vi "Predet_Inject.vi"(11 "Predet Freq (Hz)":dbl=20.0 format="%#_13g") -> ()   [LabVIEW 2017]
uses:
  <vilib>/DAQmx/write.llb/DAQmx Write (Digital 1D Wfm NChan NSamp).vi
  <vilib>/DAQmx/create/channels.llb/DAQmx Create Channel (DO-Digital Output).vi
  <vilib>/DAQmx/configure/timing.llb/DAQmx Timing (Sample Clock).vi
  <vilib>/Waveform/DWDTOps.llb/DWDT Uncompress Digital.vi
  <vilib>/DAQmx/miscellaneous.llb/DAQmx Fill In Error Info.vi
  <resource>/objmgr/daqmx.rc
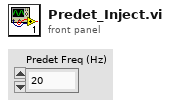
[diagram p1: front panel]
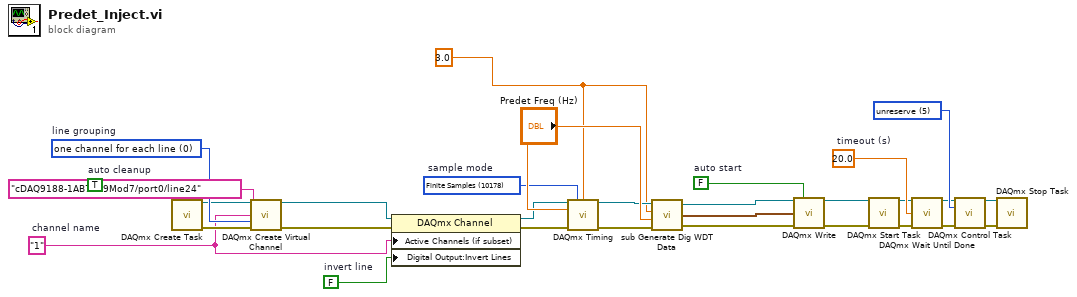
[diagram p0: block diagram]
diagram:
  w1 = 3.0 ("number of samples")
  w29 = 5 items=["verify"=2, "reserve"=4, "commit"=3, "unreserve"=5, "abort"=6] ("action")
  w20 = 10178 items=["Finite Samples"=10178, "Continuous Samples"=10123, "Hardware Timed Single Point"=12522]  # sample mode
  w18 = FALSE  # invert line
  w14 = 0 items=["one channel for each line", "one channel for all lines"]  # line grouping
  w3 = "1"  # channel name
  w12 = TRUE  # auto cleanup
  w10 = 20.0  # timeout (s)
  w4 = FALSE  # auto start
  n1 = call <vilib>:"DAQmx Create Task.vi"("auto cleanup"=w12) -> ("task out"=w13:refnum<k21>, "error out"=w11:errorcluster)  [unwired: 4 in, 9 out]
  n2 = call-poly <vilib>:"DAQmx Create Virtual Channel.vi"("task in"=w13, "lines"=tag "cDAQ9188-1AB7749Mod7/port0/line24", "name to assign"=w3, "line grouping"=w14, "error in"=w11) -> ("task out"=w15:refnum<k21>, "error out"=w16:errorcluster)  [unwired: 9 out]
  n3 = property class="DAQmx Channel"(reference=w15, error in=w16, "Active Channels (if subset)"=w3, "Digital Output:Invert Lines"=w18) -> (reference out=w19:refnum<k21>, error out=w17:errorcluster)
  n4 = call-poly <vilib>:"DAQmx Timing.vi"("task/channels in"=w19, "sample mode"=w20, "samples per channel"=w1, "rate"="Predet Freq (Hz)", "error in"=w17) -> ("task out"=w21:refnum<k21>, "error out"=w22:errorcluster)  [unwired: 2 in, 7 out]
  n5 = call <vilib>:"sub Generate Dig WDT Data.vi"("task in"=w21, "number of samples"=w1, "update rate"="Predet Freq (Hz)", "error in"=w22) -> ("task out"=w6:refnum<k21>, "data"=w9:digitalwaveform[], "error out"=w5:errorcluster)  [unwired: 1 out]
  n6 = call-poly <vilib>:"DAQmx Write.vi"("task/channels in"=w6, "auto start"=w4, "data"=w9, "error in"=w5) -> ("task out"=w24:refnum<k21>, "error out"=w23:errorcluster)  [unwired: 10 out]
  n7 = call <vilib>:"DAQmx Start Task.vi"("task/channels in"=w24, "error in"=w23) -> ("task out"=w7:refnum<k21>, "error out"=w8:errorcluster)  [unwired: 12 out]
  n8 = call <vilib>:"DAQmx Wait Until Done.vi"("task/channels in"=w7, "timeout (sec)"=w10, "error in"=w8) -> ("task out"=w25:refnum<k21>, "error out"=w28:errorcluster)  [unwired: 11 out]
  n9 = call <vilib>:"DAQmx Control Task.vi"("task/channels in"=w25, "action"=w29, "error in"=w28) -> ("task out"=w26:refnum<k21>, "error out"=w27:errorcluster)  [unwired: 11 in]
  n10 = call <vilib>:"DAQmx Stop Task.vi"("task/channels in"=w26, "error in"=w27) -> ()  [unwired: 12 in, 2 out]
